vi "Rotation.vi"() -> ()   [LabVIEW 2011]
uses:
  <vilib>/vision/NI_Vision_Development_Module.lvlib
panel:
  out "Total Frames to Rotate":u32
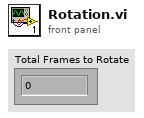
[diagram p1: front panel]
types:
  T1 = typedef "AviRefnum.ctl" = refnum<k1>
  T2 = typedef "IMAQ Image.ctl" = refnum<image>
  T3 = cluster{"width":u32, "height":u32, "framesPerSecond":u32, "compressionFilter":string, "hasData":bool}
  T4 = typedef "IMAQ Line" = cluster{"Start X":i32, "Start Y":i32, "End X":i32, "End Y":i32}
  T5 = cluster{cluster{i32, i32}, cluster{i32, i32}, cluster{"Start X":i32, "Start Y":i32}, cluster{"End X":i32, "End Y":i32}}
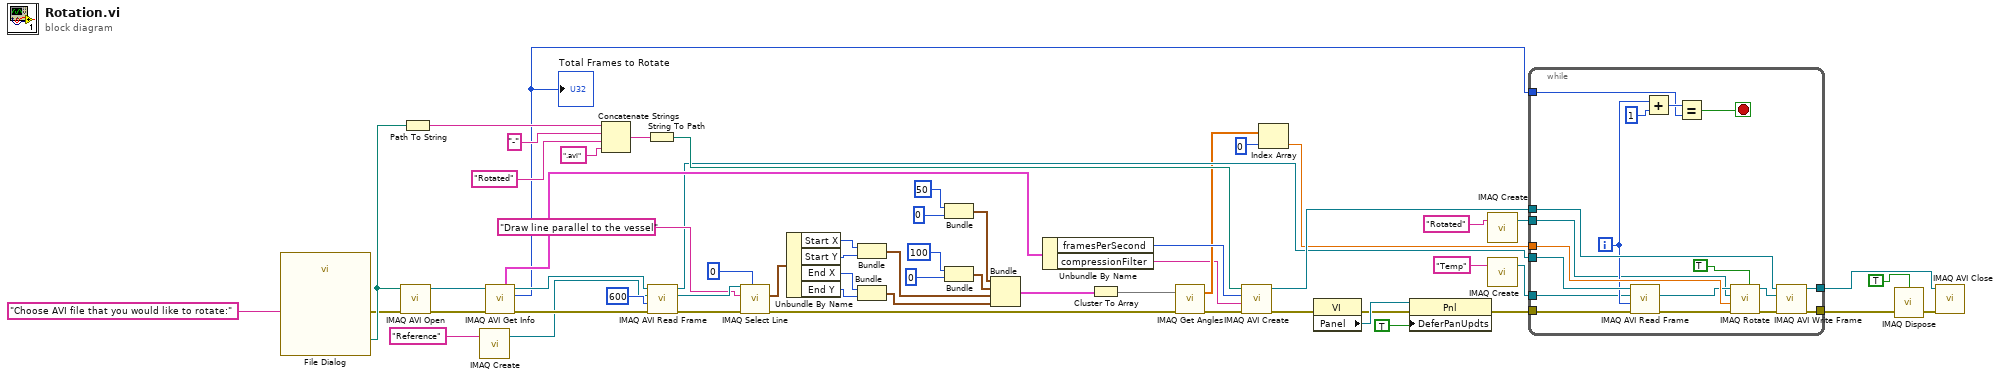
[diagram p0: block diagram]
diagram:
  n1 = call "File Dialog"("prompt"="Choose AVI file that you would like to rotate:") -> ("selected path"=w54:path, "error out"=w13:errorcluster)  [unwired: 11 in, 2 out]
  n2 = call "IMAQ AVI Open"("error in (no error)"=w13, "AVI Path"=w54) -> ("error out"=w59:errorcluster, "Avi Refnum"=w58:T1)  [unwired: 8 in]
  n3 = Path To String(path=w54) -> (string=w53:string)
  n4 = call "IMAQ Create"("Image Name"="Reference") -> ("New Image"=w42:T2)  [unwired: 4 in, 1 out]
  n5 = call "IMAQ AVI Get Info"("error in (no error)"=w59, "Avi Refnum"=w58) -> ("error out"=w45:errorcluster, "Number of Frames"=w17:u32, "Avi Refnum (duplicate)"=w44:T1, "Frame Data"=w57:T3)  [unwired: 5 in, 1 out]
  "Total Frames to Rotate" <- w17
  n6 = Concatenate Strings(w53, "-" ("string"), "Rotated" ("string"), ".avi" ("string")) -> (w50:string)
  n7 = String To Path(string=w50) -> (path=w49:path)
  n8 = call "IMAQ AVI Read Frame"("error in (no error)"=w45, "Frame Number"=u32 600, "Image"=w42, "Avi Refnum"=w44) -> ("error out"=w41:errorcluster, "Image Out"=w40:T2, "Avi Refnum (duplicate)"=w21:T1)  [unwired: 4 in, 1 out]
  n9 = call "IMAQ Select Line"("Window Number (0...15)"=0, "error in (no error)"=w41, "Prompt"="Draw line parallel to the vessel", "Image In"=w40) -> ("error out"=w22:errorcluster, "Line"=w31:T4)  [unwired: 4 in, 2 out]
  n10 = Unbundle By Name(w31) -> ("Start X"=w30:i32, "Start Y"=w29:i32, "End X"=w28:i32, "End Y"=w27:i32)
  n11 = Bundle("Start X"=w30, "Start Y"=w29) -> (w26:cluster{"Start X":i32, "Start Y":i32})  [unwired: 1 in]
  n12 = Bundle("End X"=w28, "End Y"=w27) -> (w25:cluster{"End X":i32, "End Y":i32})  [unwired: 1 in]
  n13 = Bundle(50, 0) -> (w33:cluster{i32, i32})  [unwired: 1 in]
  n14 = Bundle(100, 0) -> (w32:cluster{i32, i32})  [unwired: 1 in]
  n15 = Bundle(w33, w32, w26, w25) -> (w24:T5)  [unwired: 1 in]
  n16 = Unbundle By Name(w57) -> ("framesPerSecond"=w56:u32, "compressionFilter"=w16:string)
  n17 = Cluster To Array(cluster=w24) -> (array=w23:cluster{"End X":i32, "End Y":i32}[])
  n18 = call "IMAQ Get Angles"("error in (no error)"=w22, "Points"=w23) -> ("error out"=w15:errorcluster, "Angles (deg)"=w20:sgl[])  [unwired: 3 in, 1 out]
  n19 = call "IMAQ AVI Create"("error in (no error)"=w15, "Compression Filter"=w16, "Frames Per Second"=w56, "AVI Path"=w49) -> ("error out"=w5:errorcluster, "Avi Refnum"=w48:T1)  [unwired: 6 in]
  n20 = Index Array(array=w20, index=0) -> (element=w18:sgl)
  n21 = property class="VI"(error in=w5) -> (error out=w4:errorcluster, "Panel"=w7:refnum<vi>)  [unwired: 1 in, 1 out]
  n22 = property class="Pnl"(reference=w7, error in=w4, "DeferPanUpdts"=TRUE ("Defer Panel Updates")) -> (error out=w3:errorcluster)  [unwired: 1 out]
  n23 = call "IMAQ Create"("Image Name"="Rotated") -> ("New Image"=w9:T2)  [unwired: 4 in, 1 out]
  n24 = call "IMAQ Create"("Image Name"="Temp") -> ("New Image"=w11:T2)  [unwired: 4 in, 1 out]
  n25 = while {
    tunnel: w48 -> [w77]
    tunnel: [w76] -> w2
    tunnel: [w75] -> w47
    tunnel: w21 -> [w72]
    tunnel: w18 -> [w70]
    tunnel: w17 -> [w64]
    tunnel: w11 -> [w62]
    tunnel: w9 -> [w61]
    tunnel: w3 -> [w60]
    i -> [w67]
    stop <- w63 stop-if-true
    n26 = call "IMAQ AVI Read Frame"("error in (no error)"=w60, "Frame Number"=w67, "Image"=w62, "Avi Refnum"=w72) -> ("error out"=w73:errorcluster, "Image Out"=w69:T2)  [unwired: 4 in, 2 out]
    n27 = Add(x=w67, y=i8 1) -> (x+y=w65:i32)
    n28 = Equal?(x=w65, y=w64) -> (x = y?=w63:bool)
    n29 = call "IMAQ Rotate"("Maintain Size"=TRUE, "error in (no error)"=w73, "Angle (degrees)"=w70, "Image Dst"=w61, "Image Src"=w69) -> ("error out"=w71:errorcluster, "Image Dst Out"=w68:T2)  [unwired: 5 in]
    n30 = call "IMAQ AVI Write Frame"("error in (no error)"=w71, "Image"=w68, "Avi Refnum"=w77) -> ("error out"=w76:errorcluster, "Avi Refnum (duplicate)"=w75:T1)  [unwired: 7 in]
  }
  n31 = call "IMAQ Dispose"("All Images? (No)"=TRUE, "error in (no error)"=w2) -> ("error out"=w1:errorcluster)  [unwired: 4 in]
  n32 = call "IMAQ AVI Close"("error in (no error)"=w1, "Avi Refnum"=w47) -> ()  [unwired: 9 in, 1 out]
